vi "G#BaseClass2_Create.vi"(0 "reference in":refnum<class "G#BaseClass2.lvclass">, 1 "object name":string, 4 "no registration":bool, 5 "error in (no error)":errorcluster, 6 "create method":T1=enum."Create or look up existing", 7 "user counter":bool=TRUE) -> (14 "reference out":refnum<class "G#BaseClass2.lvclass">, 19 "error out":errorcluster)   [LabVIEW 2017, in "G#BaseClass2.lvclass"]
doc: "Constructor."
uses:
  G#BaseClass2.lvclass
  C:/Program Files/National Instruments/LabVIEW 2017/vi.lib/addons/_AddQ/G#Object/G#Object.lvclass
  <vilib>/addons/_AddQ/G#Object/utils/G#Object_CreateMethod.ctl
  <vilib>/addons/_AddQ/G#Object/G#Object.lvclass
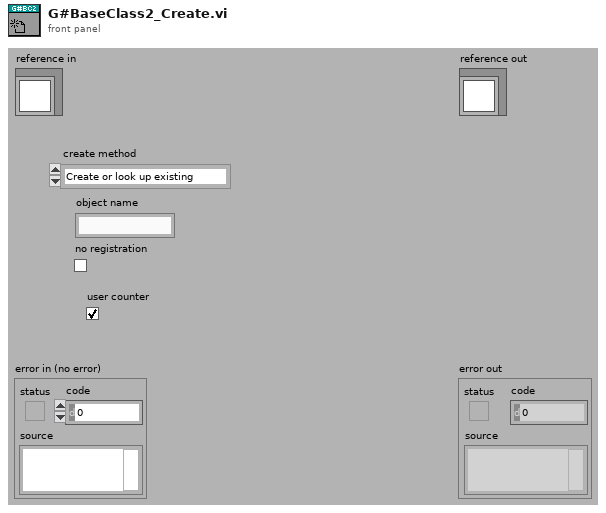
[diagram p1: front panel]
types:
  T1 = typedef "G#Object.lvclass/G#Object_CreateMethod.ctl" = enum16{"Create", "Create or look up existing", "Look up existing"}
  T2 = typedef "G#BaseClass2.lvclass/ObjectAttributes.ctl" = cluster{"Numeric":dbl, "Array":dbl[]}
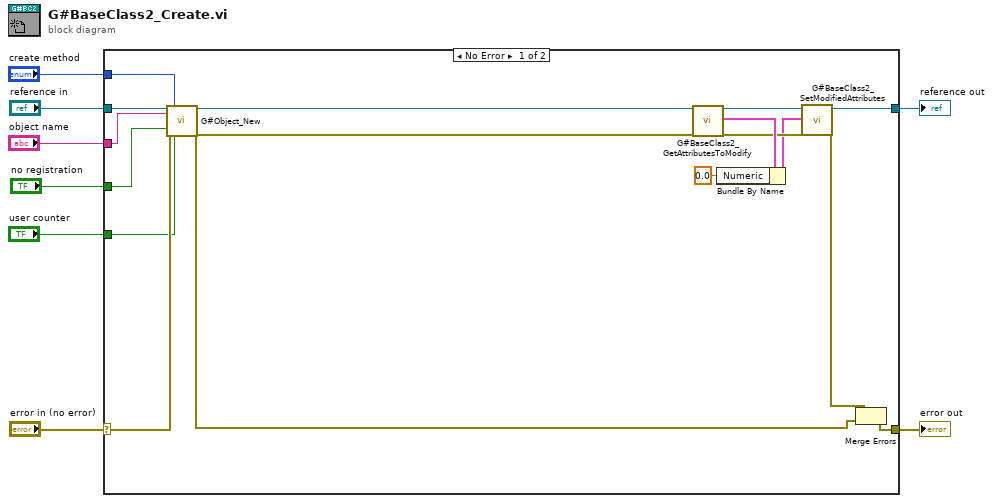
[diagram p0: block diagram]
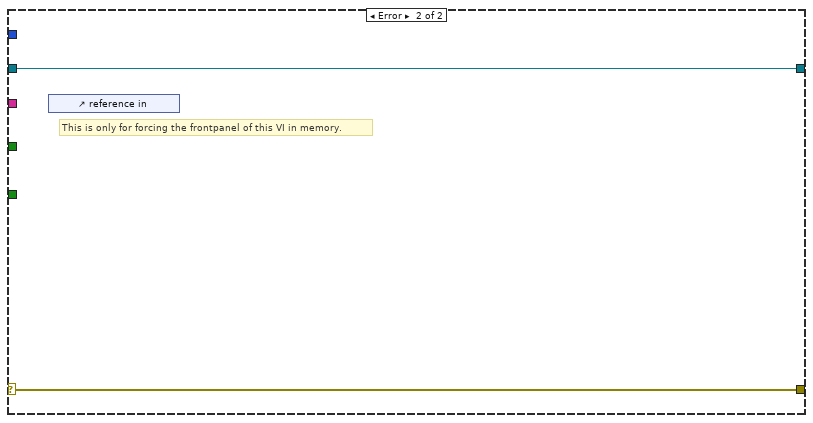
[diagram p2: hidden frame]
diagram:
  n1 = case shown="No Error" "error in (no error)" {
    selector: "error in (no error)" -> [w23 w26]
    tunnel: [w22 w26] -> w7
    tunnel: [w16 w25] -> w5
    tunnel: "reference in" -> [w24 w25]
    tunnel: "create method" -> [w12 _]
    tunnel: "object name" -> [w11 _]
    tunnel: "no registration" -> [w10 _]
    tunnel: "user counter" -> [w9 _]
    frame No Error {
      n2 = call <vilib>:"G#Object_New.vi"("reference in"=w24, "object name"=w11, "no registration? (F)"=w10, "error in (no error)"=w23, "create method"=w12, "user counter (T)?"=w9) -> ("reference out"=w21:refnum<class "G#BaseClass2.lvclass">, "error out"=w20:errorcluster)  [unwired: 11 in, 1 out]
      n3 = call "G#BaseClass2_GetAttributesToModify.vi"("reference in"=w21, "error in (no error)"=w20) -> ("reference out"=w15:refnum<class "G#BaseClass2.lvclass">, "attributes"=w19:T2, "error out"=w18:errorcluster)  [unwired: 13 in, 2 out]
      n4 = Bundle By Name(cluster=w19, "Numeric"=0.0) -> (w14:T2)
      n5 = call "G#BaseClass2_SetModifiedAttributes.vi"("reference in"=w15, "attributes"=w14, "error in (no error)"=w18) -> ("reference out"=w16:refnum<class "G#BaseClass2.lvclass">, "error out"=w17:errorcluster)  [unwired: 15 in]
      n6 = Merge Errors(w17, w20) -> (w22:errorcluster)
    }
    frame Error {
      # "This is only for forcing the frontpanel of this VI in memory."
      n7 = control-ref of="reference in"() -> ()  [unwired: 1 out]
    }
  }
  "error out" <- w7
  "reference out" <- w5
